vi "V-Meter Configure.vi"(8 "error in (no error)":errorcluster, 11 "VISA resource name in":refnum<visa-resource-name>) -> (0 "error out":errorcluster, 3 "VISA resource name out":refnum<visa-resource-name>)   [LabVIEW 2016, in "Hall Effect Library.lvlib"]
uses:
  Hall Effect Library.lvlib
  Global Variables/Instruments.vi
  V-Meter Configure (2000).vi
  V-Meter Configure (2182A).vi
  V-Meter Configure (3706).vi
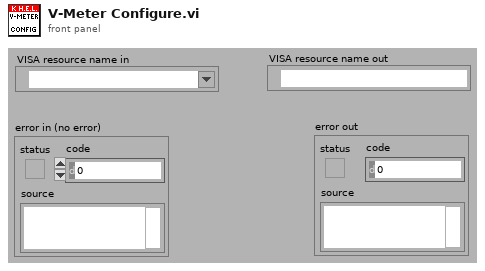
[diagram p1: front panel]
types:
  T1 = typedef "Hall Effect Library.lvlib/Voltmeters.ctl" = enum16{"2000", "2182A", "3706A"}
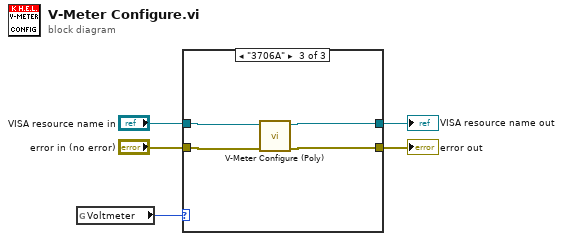
[diagram p0: block diagram]
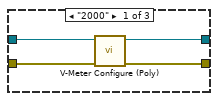
[diagram p2: hidden frame]
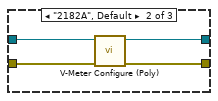
[diagram p3: hidden frame]
diagram:
  n1 = global read "Instruments.vi" "Voltmeter"() -> (w5:T1)
  n2 = case shown="\"3706A\"" w5 {
    tunnel: "VISA resource name in" -> [w9 w13 w17]
    tunnel: "error in (no error)" -> [w8 w12 w16]
    tunnel: [w7 w11 w14] -> w3
    tunnel: [w6 w10 w15] -> w4
    frame "2000" {
      n3 = call-poly "V-Meter Configure (Poly).vi"("error in (no error)"=w8, "VISA resource name in"=w9) -> ("error out"=w7:errorcluster, "VISA resource name out"=w6:refnum<visa-resource-name>)  [unwired: 8 out]
    }
    frame "2182A", Default {
      n4 = call-poly "V-Meter Configure (Poly).vi"("error in (no error)"=w12, "VISA resource name in"=w13) -> ("error out"=w11:errorcluster, "VISA resource name out"=w10:refnum<visa-resource-name>)  [unwired: 8 out]
    }
    frame "3706A" {
      n5 = call-poly "V-Meter Configure (Poly).vi"("error in (no error)"=w16, "VISA resource name in"=w17) -> ("error out"=w14:errorcluster, "VISA resource name out"=w15:refnum<visa-resource-name>)  [unwired: 8 in]
    }
  }
  "error out" <- w3
  "VISA resource name out" <- w4
